vi "ErrorHandling.ErrorToTable.vi"(11 "Errors":T1[](array[typedef])) -> (3 "Item Names":string[][](array[string]))   [LabVIEW 2016, in "ErrorHandling.lvclass"]
uses:
  ErrorHandling.lvclass
  ErrorHandling.OccurredErrorDataStruct.ctl
  <vilib>/dlg_ctls.llb/Space Constant.vi
  <vilib>/Utility/error.llb/Search and Replace Pattern.vi
  <vilib>/Utility/error.llb/Trim Whitespace.vi
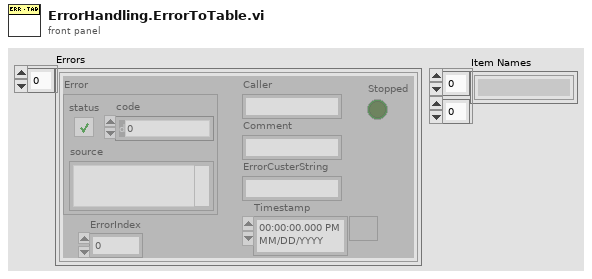
[diagram p1: front panel]
types:
  T1 = typedef "ErrorHandling.lvclass/ErrorHandling.OccurredErrorDataStruct.ctl" = cluster{"Error":errorcluster, "Caller":string, "Comment":string, "Timestamp":timestamp, "Stopped":bool, "ErrorCusterString":string, "ErrorIndex":u64}
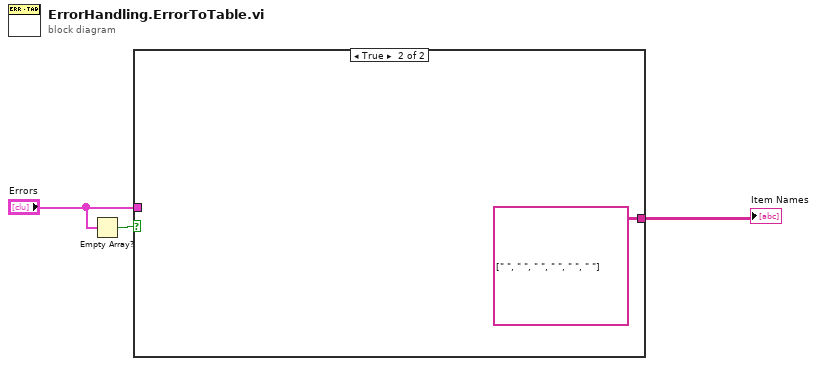
[diagram p0: block diagram]
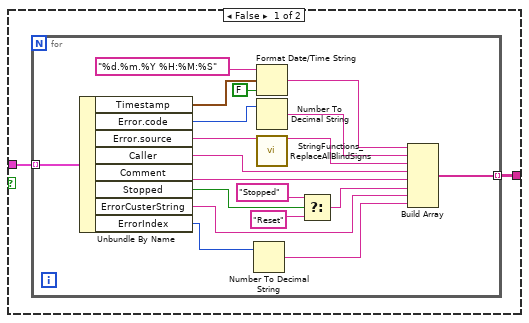
[diagram p2: hidden frame]
diagram:
  n1 = Empty Array?(array="Errors") -> (empty?=w1:bool)
  n2 = case shown="True" w1 {
    tunnel: [w5 string[][] [[" "], [" "], [" "], [" "], [" "], [" "]]] -> w3
    tunnel: "Errors" -> [w4 _]
    frame False {
      n3 = for {
        tunnel: w4 -> [w7] mode=indexing
        tunnel: [w6] -> w5 mode=indexing
        n4 = Unbundle By Name(w7) -> ("Timestamp"=w11:timestamp, "Error.code"=w8:i32, "Error.source"=w19:string, "Caller"=w21:string, "Comment"=w17:string, "Stopped"=w12:bool, "ErrorCusterString"=w22:string, "ErrorIndex"=w23:u64)
        n5 = Number To Decimal String(number=w23) -> (decimal integer string=w24:string)  [unwired: 1 in]
        n6 = Format Date/Time String(time format string (%c)="%d.%m.%Y %H:%M:%S", seconds (now)=w11, UTC format=FALSE) -> (date/time string=w15:string)
        n7 = Number To Decimal String(number=w8) -> (decimal integer string=w16:string)  [unwired: 1 in]
        n8 = call "StringFunctions_ReplaceAllBlindSigns.vi"("String"=w19) -> ("ModifiedString"=w20:string)  [unwired: 17 in, 1 out]
        n9 = Select(t="Stopped", s=w12, f="Reset") -> (s? t:f=w18:string)
        n10 = Build Array(w15, w16, w20, w21, w17, w18, w22, w24) -> (w6:string[])
      }
    }
    frame True {
    }
  }
  "Item Names" <- w3
